vi "GetImpairReports.vi"(8 "error in (no error)":errorcluster, 11 "UserPmuPlugins in":refnum<class "UserPmuImpairPlugins.lvclass">) -> (0 "error out":errorcluster, 3 "UserPmuPlugins out":refnum<class "UserPmuImpairPlugins.lvclass">)   [LabVIEW 2017, in "PmuImpairPlugins.lvlib" / "UserPmuImpairPlugins.lvclass"]
uses:
  UserPmuImpairPlugins.lvclass
  C:/Program Files (x86)/National Instruments/LabVIEW 2017/user.lib/NIST/BaseClasses/BasePlugin_class/BasePlugin.lvclass
  C:/dev/Work/PARTF/Modules/PmuImpairPlugins/PmuImpairPluginBase_class/PmuImpairPluginBase.lvclass
  <userlib>/NIST/BaseClasses/BasePlugin_class/BasePlugin.lvclass/BasePlugin.ctl
  PmuImpairPluginBase_class/PmuImpairPluginBase.lvclass/PmuImpairPluginBase.ctl
  EventPlugins/EventPluginBaseClass/TypeDefs/clEvtReport.ctl
  <userlib>/NIST/BaseClasses/BasePlugin_class/Accessors/Read PluginIniFilePath.vi
  PmuImpairPluginBase_class/Accessors/Read clEvtConfig.vi
  PmuImpairPluginBase_class/Accessors/Read BusNumber.vi
  PmuImpairPluginBase_class/Accessors/Read clImpairConfig.vi
  PmuImpairPluginBase_class/Accessors/Read dblImpairParams.vi
  <vilib>/Utility/config.llb/Read Key (String).vi
  <vilib>/Utility/config.llb/NI_LVConfig.lvlib
  EventPlugins/EventPluginBaseClass/EventPluginBaseClass.lvclass
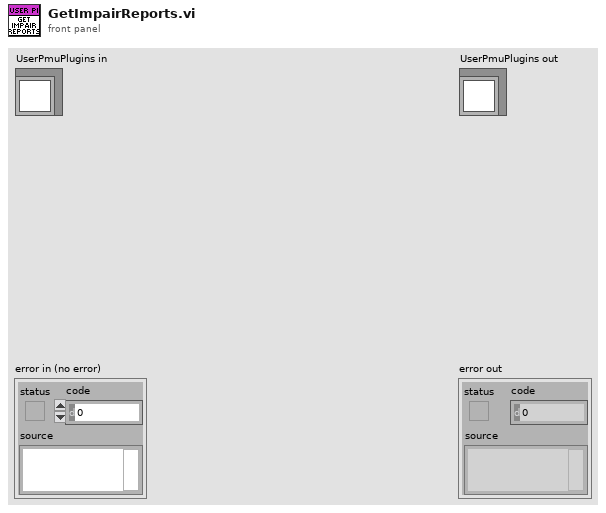
[diagram p1: front panel]
types:
  T1 = typedef "EventPlugins.lvlib/EventPluginBaseClass.lvclass/clEvtReport.ctl" = cluster{"Timestamp":dbl, "Synx":cdb[], "Freq":dbl, "ROCOF":dbl, "ID":i16}
  T2 = typedef "PmuImpairPlugins.lvlib/PmuImpairPluginBase.lvclass/clImpairConfig.ctl" = cluster{"FilterType":string, "bPosSeq":bool}
  T3 = typedef "EventPlugins.lvlib/EventPluginBaseClass.lvclass/clEvtConfig.ctl" = cluster{"T0(UTC)":dbl, "F0":dbl, "Fs":i32, "FSamp":u32, "bPosSeq":bool}
  T4 = typedef "EventPlugins.lvlib/EventPluginBaseClass.lvclass/clEvtReportArray.ctl" = T1[]
  T5 = typedef "NI_LVConfig.lvlib/Config Data RefNum.ctl" = refnum<k1>
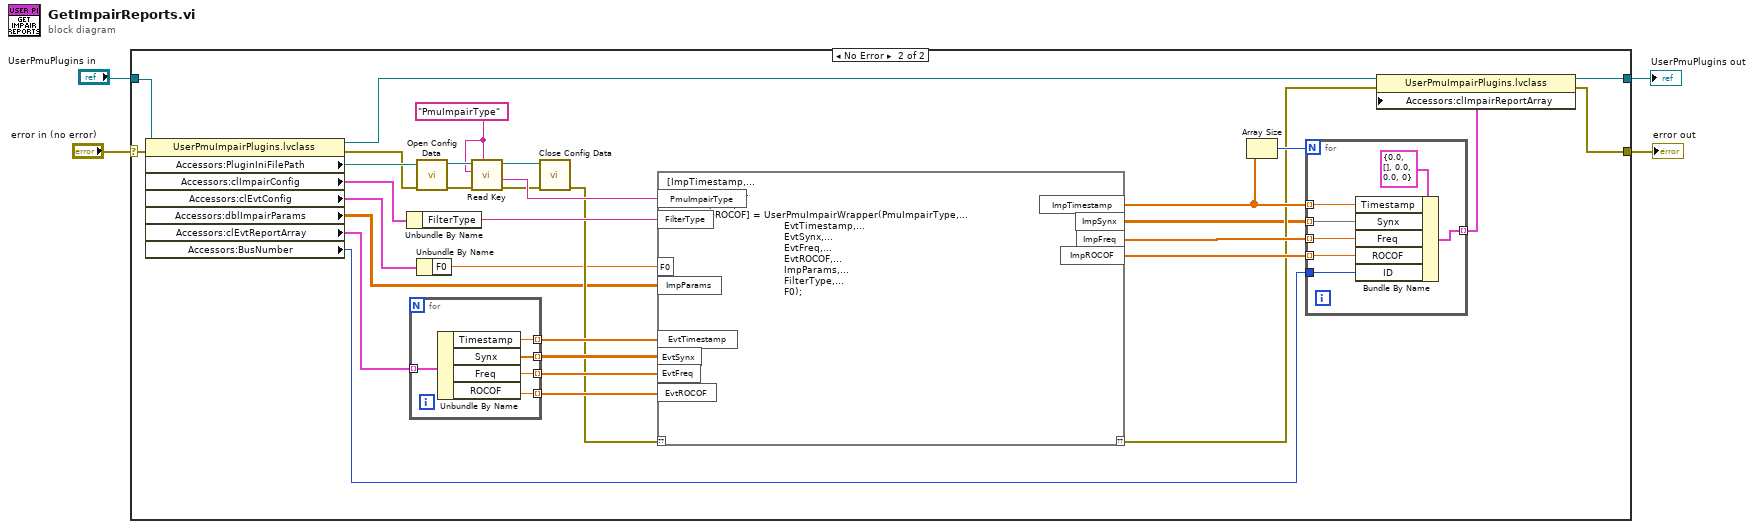
[diagram p0: block diagram]
diagram:
  n1 = case shown="No Error" "error in (no error)" {
    selector: "error in (no error)" -> [w6 w33]
    tunnel: [w5 w36] -> w1
    tunnel: "UserPmuPlugins in" -> [w5 w34]
    tunnel: [w6 w35] -> w2
    frame Error {
    }
    frame No Error {
      w16 = "PmuImpairType" ("section")
      n2 = property class="UserPmuImpairPlugins.lvclass"(reference=w34, error in=w33) -> (reference out=w32:refnum<class "UserPmuImpairPlugins.lvclass">, error out=w19:errorcluster, "Accessors:PluginIniFilePath"=w20:path, "Accessors:clImpairConfig"=w21:T2, "Accessors:clEvtConfig"=w9:T3, "Accessors:dblImpairParams"=w10:dbl[][], "Accessors:clEvtReportArray"=w11:T4, "Accessors:BusNumber"=w7:u8)
      n3 = Unbundle By Name(w21) -> ("FilterType"=w22:string)
      n4 = for {
        tunnel: w11 -> [w43] mode=indexing
        tunnel: [w42] -> w27 mode=indexing
        tunnel: [w41] -> w26 mode=indexing
        tunnel: [w40] -> w25 mode=indexing
        tunnel: [w39] -> w24 mode=indexing
        n5 = Unbundle By Name(w43) -> ("Timestamp"=w42:dbl, "Synx"=w41:cdb[], "Freq"=w40:dbl, "ROCOF"=w39:dbl)
      }
      n6 = call <vilib>:"Open Config Data.vi"("error in (no error)"=w19, "configuration file path"=w20) -> ("error out"=w18:errorcluster, "refnum"=w17:T5)  [unwired: 7 in, 1 out]
      n7 = Unbundle By Name(w9) -> ("F0"=w8:dbl)
      n8 = call-poly <vilib>:"Read Key.vi"("section"=w16, "error in (no error)"=w18, "key"=w16, "refnum"=w17) -> ("error out"=w14:errorcluster, "value"=w15:string, "refnum out"=w13:T5)  [unwired: 4 in, 1 out]
      n9 = call <vilib>:"Close Config Data.vi"("error in (no error)"=w14, "refnum"=w13) -> ("error out"=w12:errorcluster)  [unwired: 8 in, 1 out]
      n10 = script code="[ImpTimestamp,...\n          ImpSynx,...\n          ImpFreq,...\n          ImpROCOF] = UserPmuImpairWrapper(PmuImpairType,...\n                                       EvtTimestamp,...\n                                       EvtSynx,...\n                                       EvtFreq,...\n                                       EvtROCOF,...\n                                       ImpParams,...\n                                       FilterType,...\n                                       F0);"("??"=w12, "ImpParams"=w10, "FilterType"=w22, "F0"=w8, "EvtTimestamp"=w27, "EvtSynx"=w26, "EvtFreq"=w25, "EvtROCOF"=w24, "PmuImpairType"=w15) -> ("??"=w29:errorcluster, "ImpTimestamp"=w31:dbl[], "ImpSynx"=w28:cdb[][], "ImpFreq"=w38:dbl[], "ImpROCOF"=w37:dbl[])
      n11 = Array Size(array=w31) -> (size(s)=w30:i32)
      n12 = for {
        N: w30 -> [_]
        tunnel: w31 -> [w50] mode=indexing
        tunnel: w38 -> [w49] mode=indexing
        tunnel: w37 -> [w48] mode=indexing
        tunnel: w28 -> [w47] mode=indexing
        tunnel: [w45] -> w23 mode=indexing
        tunnel: w7 -> [w44]
        n13 = Bundle By Name(cluster=T1 {"Timestamp"=0.0, "Synx"=[], "Freq"=0.0, "ROCOF"=0.0, "ID"=0} ("clEvtReport"), "Timestamp"=w50, "Synx"=w47, "Freq"=w49, "ROCOF"=w48, "ID"=w44) -> (w45:T1)
      }
      n14 = property class="UserPmuImpairPlugins.lvclass"(reference=w32, error in=w29, "Accessors:clImpairReportArray"=w23) -> (reference out=w36:refnum<class "UserPmuImpairPlugins.lvclass">, error out=w35:errorcluster)
    }
  }
  "error out" <- w2
  "UserPmuPlugins out" <- w1
